vi "Temperature Warnings.vi"(8 "Error In":errorcluster, 11 "Cluster":T1) -> (0 "Error Out":errorcluster, 1 "Cluster 2":T1, 2 "standard warning":string, 3 "Warning?":bool)   [LabVIEW 2025]
doc: "This VI is used to determine the string to output to the weather station based on the current temperature and limit settings.\n\nInputs: Current Temperature (DBL), Minimum Temperature (DBL), and Maximum Temperature (DBL).\nOutputs: Warning Text (string) and Warning? (Boolean)."
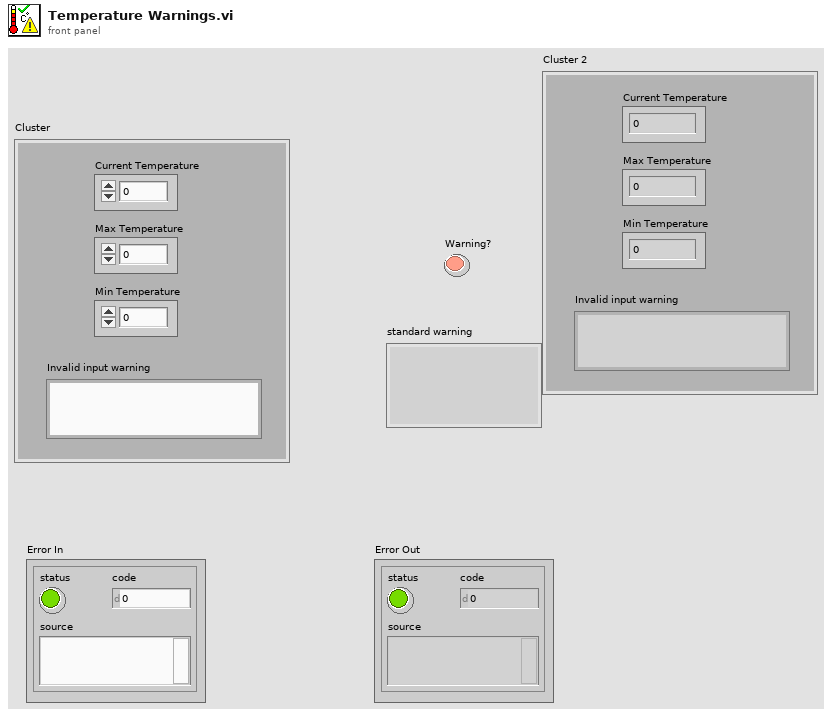
[diagram p1: front panel]
types:
  T1 = cluster{"Current Temperature":dbl, "Max Temperature":dbl, "Min Temperature":dbl, "Invalid input warning":string}
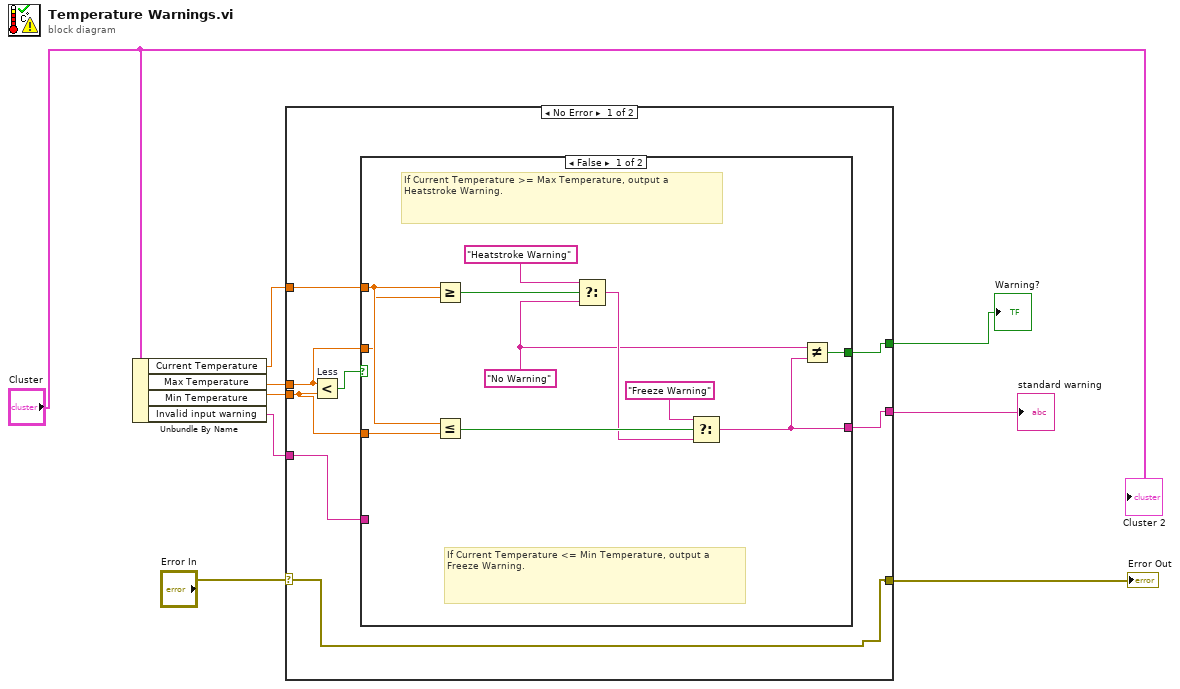
[diagram p0: block diagram]
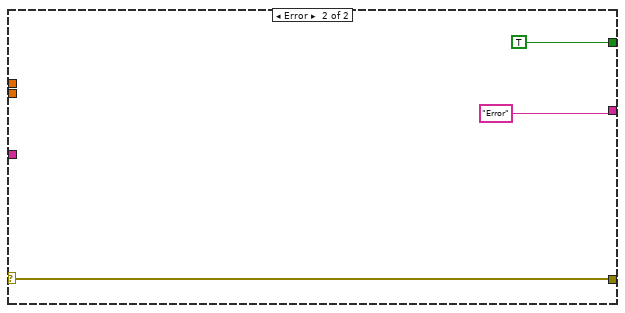
[diagram p3: hidden frame]
diagram:
  n1 = Unbundle By Name("Cluster") -> ("Current Temperature"=w6:dbl, "Max Temperature"=w8:dbl, "Min Temperature"=w7:dbl, "Invalid input warning"=w1:string)
  n2 = case shown="No Error" "Error In" {
    selector: "Error In" -> [w10 w32]
    tunnel: [w10 w32] -> w9
    tunnel: w8 -> [w13 _]
    tunnel: w7 -> [w12 _]
    tunnel: w6 -> [w16 _]
    tunnel: [w15 TRUE] -> w4
    tunnel: [w14 "Error"] -> w3
    tunnel: w1 -> [w11 _]
    frame No Error {
      n3 = Less? "Less"(x=w13, y=w12) -> (x < y?=w17:bool)
      n4 = case shown="False" w17 {
        selector: w17 -> [_ w29]
        tunnel: w16 -> [w28 _]
        tunnel: w12 -> [w27 _]
        tunnel: w13 -> [w26 _]
        tunnel: [w25 w29] -> w15
        tunnel: [w24 w30] -> w14
        tunnel: w11 -> [_ w30]
        frame False {
          w18 = "No Warning" ("f")
          # "If Current Temperature >= Max Temperature, output a Heatstroke Warning."
          # "If Current Temperature <= Min Temperature, output a Freeze Warning."
          n5 = Greater Or Equal?(x=w28, y=w26) -> (x >= y?=w23:bool)
          n6 = Less Or Equal?(x=w28, y=w27) -> (x <= y?=w20:bool)
          n7 = Select(t="Heatstroke Warning", s=w23, f=w18) -> (s? t:f=w19:string)
          n8 = Select(t="Freeze Warning", s=w20, f=w19) -> (s? t:f=w24:string)
          n9 = Not Equal?(x=w18, y=w24) -> (x != y?=w25:bool)
        }
        frame True {
        }
      }
    }
    frame Error {
    }
  }
  "Error Out" <- w9
  "Warning?" <- w4
  "standard warning" <- w3
  "Cluster 2" <- "Cluster"
